vi "auto_detect_arduino.vi"(0 "instr name":string="Arduino" caption="Arduino Board Name", 1 "error in":errorcluster) -> (2 "VISA resource name":refnum<visa-resource-name>, 3 "status":bool, 4 "error out":errorcluster)   [LabVIEW 2014]
uses:
  <vilib>/Instr/_visa.llb/VISA Find Search Mode.ctl
  <vilib>/regexp/Match Regular Expression.xnode
panel:
  # "Auto Detect ARDUINO"
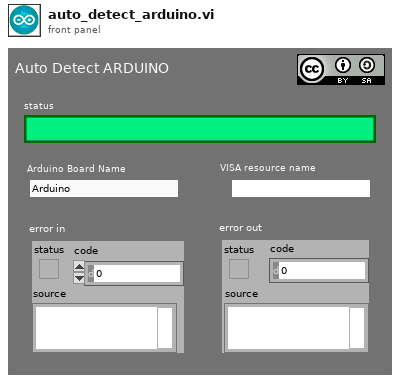
[diagram p1: front panel]
types:
  T1 = typedef "VISA Find Search Mode.ctl" = u32
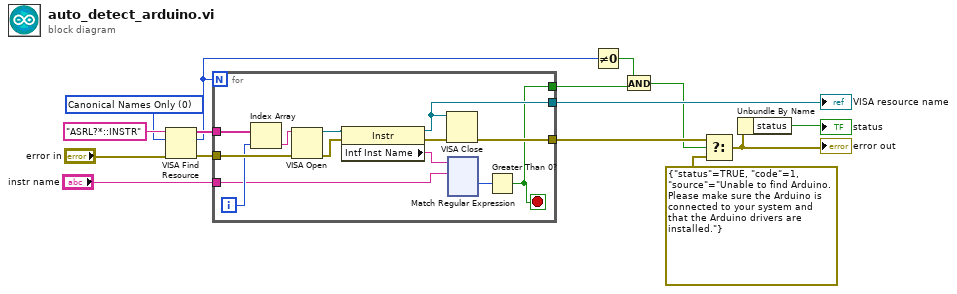
[diagram p0: block diagram]
diagram:
  w4 = T1 0 items=["Canonical Names Only"=0, "Aliases Only"=2, "Include Matching Aliases"=3, "Include All Aliases"=4] ("Search Mode")
  n1 = VISA Find Resource(8:"error in", 10:w4, 11:"ASRL?*::INSTR" ("expression (\"?*\")")) -> (0:w6:errorcluster, 2:w5:u32, 3:w7:string[])
  n2 = for {
    N: w5 -> [_]
    tunnel: w7 -> [w28]
    tunnel: w6 -> [w27]
    tunnel: [w19] -> w10
    tunnel: [w26] -> w15
    tunnel: "instr name" -> [w17]
    tunnel: [w16] -> w3
    i -> [w25]
    stop <- w16 stop-if-true
    n3 = Index Array(array=w28, index=w25) -> (element=w24:string)
    n4 = VISA Open(error in (no error)=w27, VISA resource name=w24) -> (VISA resource name=w23:refnum<visa-resource-name>, error out=w22:errorcluster)  [unwired: 3 in]
    n5 = property class="Instr"(reference=w23, error in=w22) -> (reference out=w19:refnum<visa-resource-name>, error out=w21:errorcluster, "Intf Inst Name"=w18:string)
    n6 = VISA Close(VISA resource name=w19, error in (no error)=w21) -> (error out=w26:errorcluster)
    n7 = xnode "Match Regular Expression"("input string"=w18, "regular expression"=w17) -> ("offset past match"=w20:i32)  [unwired: 4 in, 4 out]
    n8 = Greater Than 0?(x=w20) -> (x > 0?=w16:bool)
  }
  "VISA resource name" <- w10
  n9 = Not Equal To 0?(x=w5) -> (x != 0?=w2:bool)
  n10 = And(x=w2, y=w3) -> (x .and. y?=w1:bool)
  n11 = Select(t=w15, s=w1, f=errorcluster {"status"=TRUE, "code"=1, "source"="Unable to find Arduino.  Please make sure the Arduino is connected to your system and that the Arduino drivers are installed."}) -> (s? t:f=w13:errorcluster)
  "error out" <- w13
  n12 = Unbundle By Name(w13) -> ("status"=→"status":bool)
